vi "Delete Child.vi"(8 "error in (no error)":errorcluster, 9 "Position":i32[](array[numeric]), 10 "Tree In":refnum<class "Tree.lvclass">, 11 "Composite Tree Data in":refnum<class "Composite Tree Data.lvclass">) -> (0 "error out":errorcluster, 1 "Delete Child Out":refnum<class "Tree Data.lvclass">, 2 "Tree Out":refnum<class "Tree.lvclass">, 3 "Composite Tree Data out":refnum<class "Composite Tree Data.lvclass">)   [LabVIEW 2022 SP3, in "Composite Tree Data.lvclass"]
uses:
  Composite Tree Data.lvclass
  C:/Users/User/Desktop/Bussiness/Tricorn Re/Mandelbrot 4.0/General Library V2/Ancestor Class/Front Panel Container/Tree/Tree Data/Tree Data.lvclass
  Tree/Tree.lvclass
  Tree Data/Tree Data.lvclass
  Tree Data/Tree Data.lvclass/Tree Data.ctl
  Composite Tree Data.lvclass/Composite Tree Data.ctl
  Tree/Public Data/Read Root Tag.vi
  Tree Data/Protected Data/Read Tag.vi
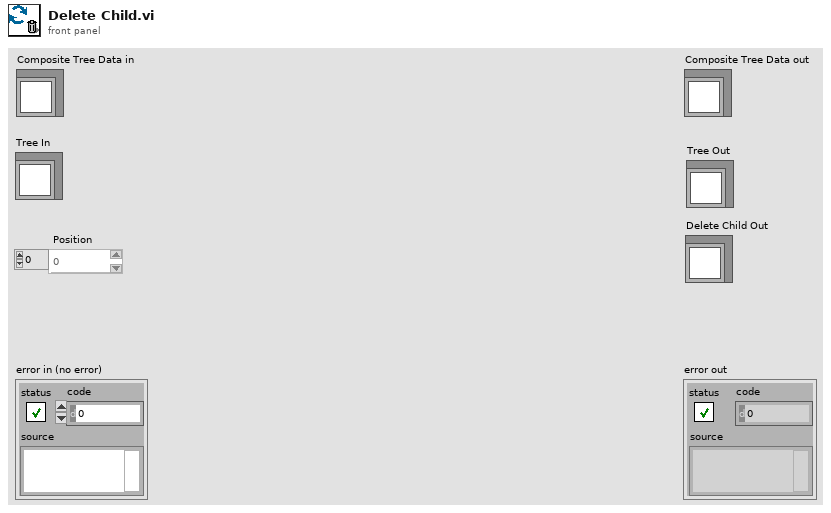
[diagram p1: front panel]
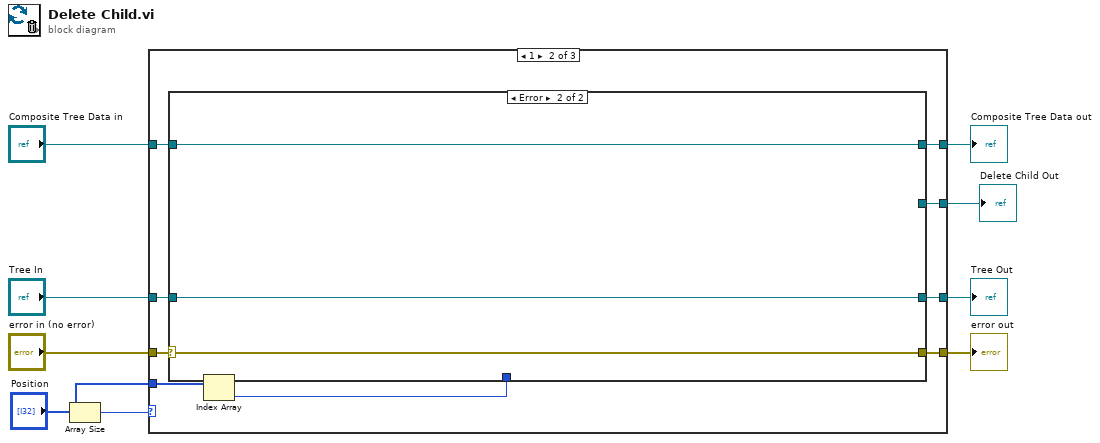
[diagram p0: block diagram]
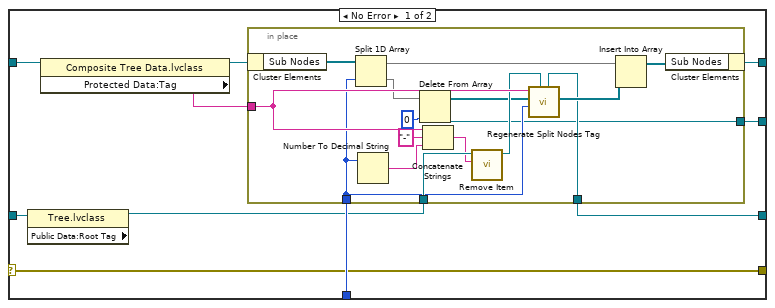
[diagram p3: hidden frame]
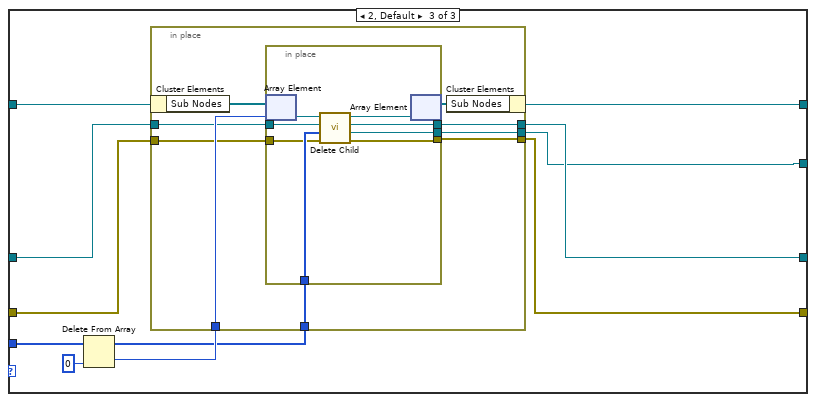
[diagram p4: hidden frame]
diagram:
  n1 = Array Size(array="Position") -> (size(s)=w3:i32)
  n2 = case shown="1" w3 {
    tunnel: "error in (no error)" -> [w10 w21 w55]
    tunnel: [w10 w20 w52] -> w8
    tunnel: "Composite Tree Data in" -> [w12 w19 w58]
    tunnel: [w12 w18 w57] -> w6
    tunnel: [w11 w17 w53] -> w5
    tunnel: "Tree In" -> [w11 w16 w56]
    tunnel: "Position" -> [_ w15 w54]
    tunnel: [_ w13 w51] -> w1
    frame 0 {
    }
    frame 1 {
      n3 = Index Array(array=w15) -> (element=w14:i32)  [unwired: 1 in]
      n4 = case shown="Error" w21 {
        selector: w21 -> [w23 w50]
        tunnel: [w23 w50] -> w20
        tunnel: [w28 w49] -> w18
        tunnel: w19 -> [w27 w49]
        tunnel: [w24 w48] -> w17
        tunnel: w16 -> [w31 w48]
        tunnel: w14 -> [w30 _]
        tunnel: [w22 _] -> w13
        frame No Error {
          n5 = property class="Tree.lvclass" props=["Public Data:Root Tag"](reference=w31) -> (reference out=w29:refnum<class "Tree.lvclass">)  [unwired: 1 in, 2 out]
          n6 = property class="Composite Tree Data.lvclass"(reference=w27) -> (reference out=w26:refnum<class "Composite Tree Data.lvclass">, "Protected Data:Tag"=w25:string)  [unwired: 1 in, 1 out]
          n7 = in-place {
            in-place-border: w30 -> [w36]
            in-place-border: w29 -> [w46]
            in-place-border: w25 -> [w41]
            in-place-border: [w37] -> w24
            in-place-border: [w32] -> w22
            n8 = in-place-cluster #1(w26) -> ("Sub Nodes"=w47:refnum<class "Tree Data.lvclass">[])
            n9 = Split 1D Array(array=w47, index=w36) -> (first subarray=w45:refnum<class "Tree Data.lvclass">[], second subarray=w35:refnum<class "Tree Data.lvclass">[])
            n10 = Number To Decimal String(number=w36) -> (decimal integer string=w43:string)  [unwired: 1 in]
            n11 = Delete From Array(array=w35, index=0) -> (deleted portion=w32:refnum<class "Tree Data.lvclass">, array with subset deleted=w33:refnum<class "Tree Data.lvclass">[])  [unwired: 1 in]
            n12 = Concatenate Strings(w41, "-" ("string"), w43) -> (w42:string)
            n13 = call "Remove Item.vi"("Tag In"=w42, "Tree in"=w46) -> ("Tree out"=w40:refnum<class "Tree.lvclass">)  [unwired: 8 in, 1 out]
            n14 = call "Regenerate Split Nodes Tag.vi"("Tree In"=w40, "Start Index"=w36, "Split Node In"=w33, "Parent Tag In"=w41) -> ("Split Node Out"=w39:refnum<class "Tree Data.lvclass">[], "Tree Out"=w37:refnum<class "Tree.lvclass">)  [unwired: 5 in, 1 out]
            n15 = Insert Into Array(array=w45, new element=w39) -> (w38:refnum<class "Tree Data.lvclass">[])  [unwired: 1 in]
            n16 = in-place-cluster #1("Sub Nodes"=w38) -> (w28:refnum<class "Composite Tree Data.lvclass">)
          }
        }
        frame Error {
        }
      }
    }
    frame 2, Default {
      n17 = Delete From Array(array=w54, index=0) -> (deleted portion=w60:i32, array with subset deleted=w59:i32[])  [unwired: 1 in]
      n18 = in-place {
        in-place-border: w60 -> [w69]
        in-place-border: w56 -> [w67]
        in-place-border: w55 -> [w66]
        in-place-border: w59 -> [w65]
        in-place-border: [w64] -> w53
        in-place-border: [w63] -> w52
        in-place-border: [w62] -> w51
        n19 = in-place-cluster #2(w58) -> ("Sub Nodes"=w70:refnum<class "Tree Data.lvclass">[])
        n20 = in-place {
          in-place-border: w67 -> [w75]
          in-place-border: w66 -> [w74]
          in-place-border: w65 -> [w76]
          in-place-border: [w73] -> w64
          in-place-border: [w72] -> w63
          in-place-border: [w71] -> w62
          n21 = in-place-array #3(w70, w69) -> (w78:refnum<class "Tree Data.lvclass">)
          n22 = call-dynamic "Delete Child.vi"("error in (no error)"=w74, "Position"=w76, "Tree In"=w75, "Tree Data in"=w78) -> ("error out"=w72:errorcluster, "Delete Child Out"=w71:refnum<class "Tree Data.lvclass">, "Tree Out"=w73:refnum<class "Tree.lvclass">, "Tree Data out"=w77:refnum<class "Tree Data.lvclass">)  [unwired: 4 in]
          n23 = in-place-array #3(w77) -> (w68:refnum<class "Tree Data.lvclass">[])  [unwired: 1 out]
        }
        n24 = in-place-cluster #2("Sub Nodes"=w68) -> (w57:refnum<class "Composite Tree Data.lvclass">)
      }
    }
  }
  "error out" <- w8
  "Composite Tree Data out" <- w6
  "Tree Out" <- w5
  "Delete Child Out" <- w1
